vi "CRYAuto Create Recalled Curves.vi"(8 "all or last":i32, 9 "Curve Names in":string[](array[string]), 10 "Curves Selected?":bool[](array[boolean]), 11 "Data Array":T1[](array[typedef]) {"Z data" items=["dB", "Lin"]; "X data" items=["dB", "Lin"]; "Y data" items=["dB", "Lin"]; "Z dB ref" format="%.1f"; "Z axis" items=["Log", "Lin"]; "X dB ref" format="%.1f"; "X axis" items=["Log", "Lin"]; "Y axis" items=["Log", "Lin"]; "Y dB ref" format="%.1f"; "Curve"."z" format="%.2f"; "Curve"."y" format="%.2f"; "Curve"."x" format="%.2f"}) -> (3 "Data Out":T1[](array[typedef]) {"Z data" items=["dB", "Lin"]; "X data" items=["dB", "Lin"]; "Y data" items=["dB", "Lin"]; "Z dB ref" format="%.1f"; "Z axis" items=["Log", "Lin"]; "X dB ref" format="%.1f"; "X axis" items=["Log", "Lin"]; "Y axis" items=["Log", "Lin"]; "Y dB ref" format="%.1f"; "Curve"."z" format="%.2f"; "Curve"."y" format="%.2f"; "Curve"."x" format="%.2f"})   [LabVIEW 2013]
uses:
  Typedef Control/CRYData Cluster.ctl
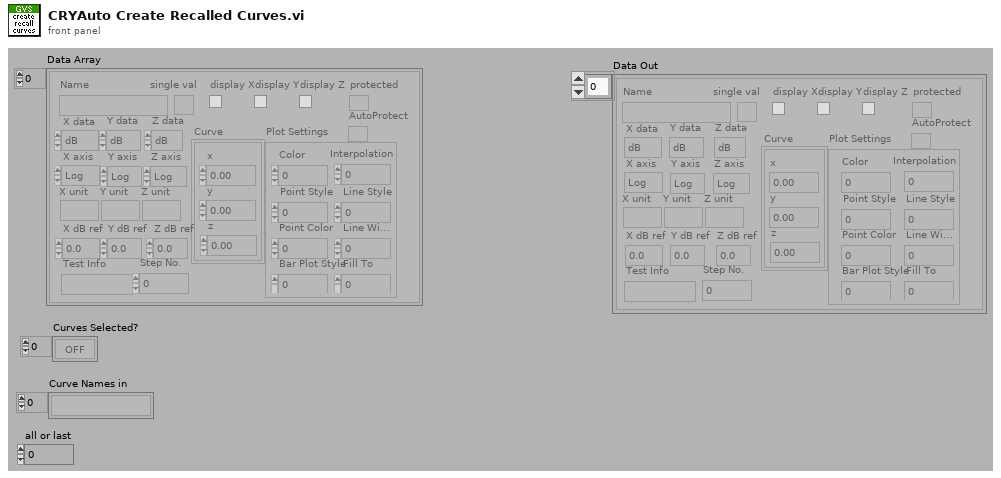
[diagram p1: front panel]
types:
  T1 = typedef "CRYData Cluster.ctl" = cluster{"Name":string, "Curve":cluster{"x":dbl, "y":dbl, "z":dbl}[], "X data":u16, "Y data":u16, "Z data":u16, "X axis":u16, "Y axis":u16, "Z axis":u16, "X unit":string, "Y unit":string, "Z unit":string, "X dB ref":dbl, "Y dB ref":dbl, "Z dB ref":dbl, "single val":bool, "protected":bool, "display X":bool, "display Y":bool, "display Z":bool, "Test Info":string, "Step No.":i32, "Plot Settings":cluster{"Color":u32, "Interpolation":u8, "Point Style":u8, "Line Style":u8, "Point Color":u32, "Line Width":u8, "Bar Plot Style":u8, "Fill To":i16}, "AutoProtect":bool}
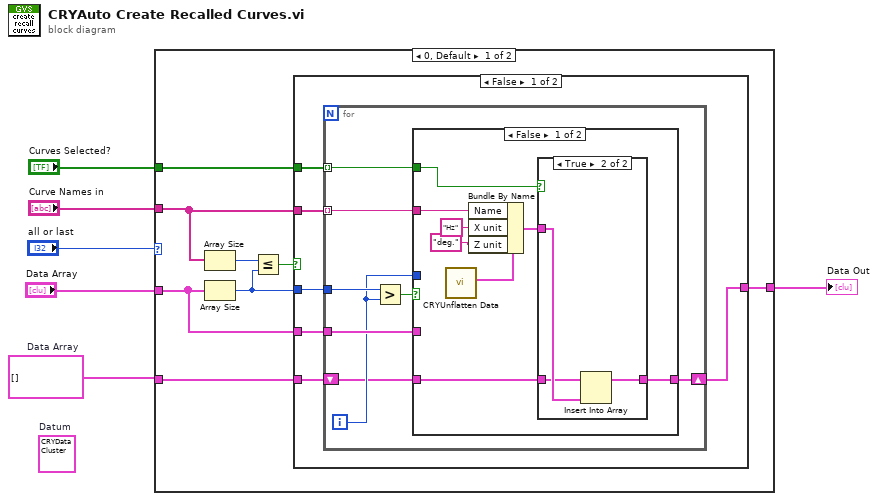
[diagram p0: block diagram]
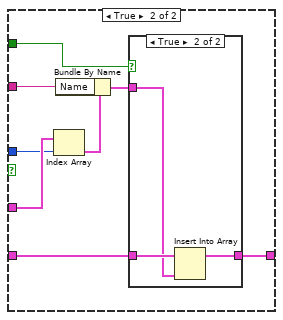
[diagram p3: hidden frame]
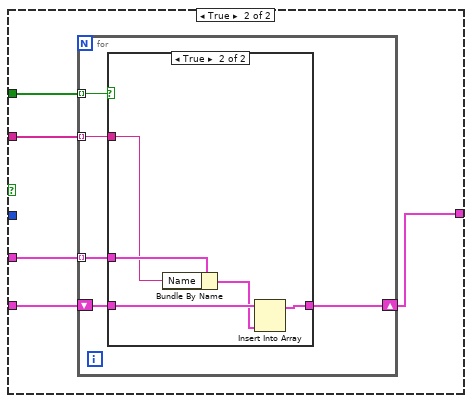
[diagram p5: hidden frame]
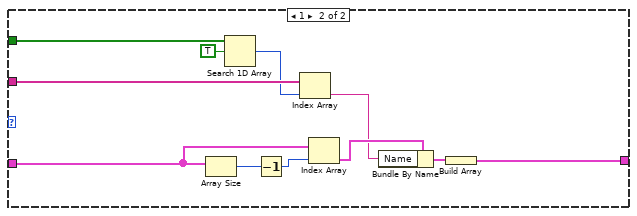
[diagram p7: hidden frame]
diagram:
  (unwired) T1 {"Name"="", "Curve"=[], "X data"=0, "Y data"=0, "Z data"=0, "X axis"=0, "Y axis"=0, "Z axis"=0, "X unit"="", "Y unit"="", "Z unit"="", "X dB ref"=0.0, "Y dB ref"=0.0, "Z dB ref"=0.0, "single val"=FALSE, "protected"=FALSE, "display X"=FALSE, "display Y"=FALSE, "display Z"=FALSE, "Test Info"="", "Step No."=0, "Plot Settings"={"Color"=0, "Interpolation"=0, "Point Style"=0, "Line Style"=0, "Point Color"=0, "Line Width"=0, "Bar Plot Style"=0, "Fill To"=0}, "AutoProtect"=FALSE}  # Datum
  w1 = T1[] []  # Data Array
  n1 = case shown="0, Default" "all or last" {
    tunnel: "Data Array" -> [w11 w74]
    tunnel: "Curve Names in" -> [w9 w77]
    tunnel: "Curves Selected?" -> [w12 w79]
    tunnel: [w8 w69] -> w2
    tunnel: w1 -> [w10 _]
    frame 0, Default {
      n2 = Array Size(array=w9) -> (size(s)=w14:i32)
      n3 = Array Size(array=w11) -> (size(s)=w7:i32)
      n4 = Less Or Equal?(x=w14, y=w7) -> (x <= y?=w13:bool)
      n5 = case shown="False" w13 {
        tunnel: w12 -> [w20 w57]
        tunnel: w11 -> [w17 w56]
        tunnel: w10 -> [w16 w55]
        tunnel: w9 -> [w19 w53]
        tunnel: [w15 w54] -> w8
        tunnel: w7 -> [w18 _]
        frame False {
          n6 = for {
            tunnel: w20 -> [w26] mode=indexing
            tunnel: w19 -> [w23] mode=indexing
            tunnel: w18 -> [w28]
            tunnel: w17 -> [w25]
            shift-right: [w21] -> w15
            shift-left: w16 -> [w22]
            i -> [w24]
            n7 = Greater?(x=w28, y=w24) -> (0:w27:bool)
            n8 = case shown="False" w27 {
              tunnel: w26 -> [w36 w48]
              tunnel: w25 -> [_ w47]
              tunnel: w24 -> [_ w46]
              tunnel: w23 -> [w34 w44]
              tunnel: w22 -> [w30 w42]
              tunnel: [w29 w41] -> w21
              frame False {
                n9 = call "CRYUnflatten Data.vi"() -> ("Datum"=w35:T1)  [unwired: 9 in, 2 out]
                n10 = Bundle By Name(cluster=w35, "Name"=w34, "X unit"="Hz", "Z unit"="deg.") -> (w31:T1)
                n11 = case shown="True" w36 {
                  tunnel: w31 -> [_ w40]
                  tunnel: w30 -> [w37 w39]
                  tunnel: [w37 w38] -> w29
                  frame False {
                  }
                  frame True {
                    n12 = Insert Into Array(array=w39, new element=w40) -> (w38:T1[])  [unwired: 1 in]
                  }
                }
              }
              frame True {
                n13 = Index Array(array=w47, index=w46) -> (element=w45:T1)
                n14 = Bundle By Name(cluster=w45, "Name"=w44) -> (w43:T1)
                n15 = case shown="True" w48 {
                  tunnel: w43 -> [_ w51]
                  tunnel: w42 -> [w49 w52]
                  tunnel: [w49 w50] -> w41
                  frame False {
                  }
                  frame True {
                    n16 = Insert Into Array(array=w52, new element=w51) -> (w50:T1[])  [unwired: 1 in]
                  }
                }
              }
            }
          }
        }
        frame True {
          n17 = for {
            tunnel: w57 -> [w62] mode=indexing
            tunnel: w56 -> [w59] mode=indexing
            shift-right: [w60] -> w54
            shift-left: w55 -> [w61]
            tunnel: w53 -> [w58] mode=indexing
            n18 = case shown="True" w62 {
              tunnel: w59 -> [_ w66]
              tunnel: w61 -> [w63 w68]
              tunnel: [w63 w67] -> w60
              tunnel: w58 -> [_ w65]
              frame False {
              }
              frame True {
                n19 = Bundle By Name(cluster=w66, "Name"=w65) -> (w64:T1)
                n20 = Insert Into Array(array=w68, new element=w64) -> (w67:T1[])  [unwired: 1 in]
              }
            }
          }
        }
      }
    }
    frame 1 {
      n21 = Array Size(array=w74) -> (size(s)=w75:i32)
      n22 = Search 1D Array(1D array=w79, element=TRUE) -> (index of element=w76:i32)  [unwired: 1 in]
      n23 = Decrement(x=w75) -> (x-1=w73:i32)
      n24 = Index Array(array=w77, index=w76) -> (element=w71:string)
      n25 = Index Array(array=w74, index=w73) -> (element=w72:T1)
      n26 = Bundle By Name(cluster=w72, "Name"=w71) -> (w70:T1)
      n27 = Build Array(w70) -> (w69:T1[])
    }
  }
  "Data Out" <- w2
